vi "V-Meter Zero (2000).vi"(8 "error in (no error)":errorcluster, 11 "VISA resource name in":refnum<visa-resource-name>) -> (0 "error out":errorcluster, 3 "VISA resource name out":refnum<visa-resource-name>)   [LabVIEW 2016, in "Hall Effect Library.lvlib"]
uses:
  Hall Effect Library.lvlib
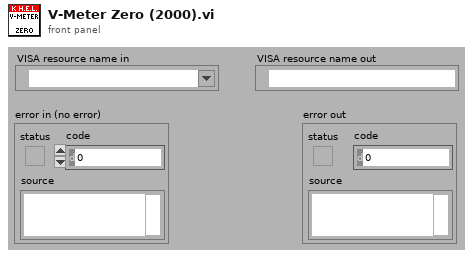
[diagram p1: front panel]
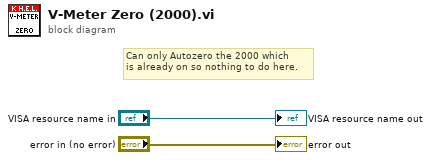
[diagram p0: block diagram]
diagram:
  # "Can only Autozero the 2000 which\nis already on so nothing to do here."
  "error out" <- "error in (no error)"
  "VISA resource name out" <- "VISA resource name in"
